vi "CSHostTest.vi"() -> ()   [LabVIEW 2014]
uses:
  <vilib>/FPGAPlugInAG/PXI-7852R/niLvFpga_Open_PXI-7852R.vi
  <vilib>/rvi/interface/common/dynamic/niFpgaDynamicAddResources.vi
  <vilib>/rvi/interface/common/niFpgaWaitOnOcc.vi
  <vilib>/Utility/error.llb/Error Cluster From Error Code.vi
  <vilib>/rvi/errors/niLvFpgaAdjustHostInterfaceError.vi
  <vilib>/FPGAPlugInAG/Dynamic/niLvFpga_Close_Dynamic.vi
  <vilib>/rvi/interface/nirviOpenFPGA/nirviOpenFPGA.xnode
  FPGA Bitfiles/TiTaProj_DAF_sequencerCWTopLevel_102.lvbitx
  <vilib>/rvi/interface/nirviMethod/nirviMethod.xnode
  <vilib>/rvi/interface/nirviReadWriteControl/nirviReadWriteControl.xnode
  <vilib>/rvi/interface/nirviCloseFPGA/nirviCloseFPGA.xnode
  <vilib>/rvi/interface/Simulation/niFpgaSimulationCallBeginRW.vi
  <vilib>/FPGAPlugInAG/Dynamic/niLvFpga_ReadFifo_Dynamic.vi
  <vilib>/rvi/errors/niLvFpgaMergeErrorWithErrorCode.vi
  NiFpgaLv.dll
  <vilib>/FPGAPlugInAG/Dynamic/niLvFpga_ConfigureFifo_Dynamic.vi
panel:
  in  "SendCommand":bool
  out "SavedData":u32[](array[numeric]) format="%032b"
  out "CounterArray":u32[][][](array[numeric])
  out "VoltArray":u32[](array[numeric]) format="%032b"
  in  "AnalyseData":bool
  in  "dwellTime":u32=2000000
  out "ReadData":u32[](array[numeric]) format="%032b"
  in  "stop":bool
  in  "abort":bool
  in  "hostConfirmsHzOffsetIsSet":bool
  in  "halt":bool
  in  "SetParameters":bool
  in  "VoltOrScaler?":bool
  in  "stepSize":i32=32768 format="%024b"
  in  "start":i32 format="%024b"
  in  "nOfSteps":i32=20
  in  "nOfScans":i32=6
  in  "invertScan":bool
  in  "heinzingerControl":T1(ring)
  in  "waitForKepco(25nsTicks)":u16
  in  "waitAfterReset(25nsTicks)":u16
  in  "measVoltPulseLength(25ns)":i32
  in  "measVoltTimeout(10ns)":i32
  in  "cmdByHost":T2(ring)
  out "measVoltState":T3(ring)
  out "seqState":T2(ring)
  out "SCstate":enum16{"idle", "scanning", "done", "error"}(ring)
  out "SCerrorcount":u8
  out "DACQuWriteTimeout":bool
  out "SCQuWriteTimeout":bool
  # "Scan"
  # "nOfPMT"
  # "Step"
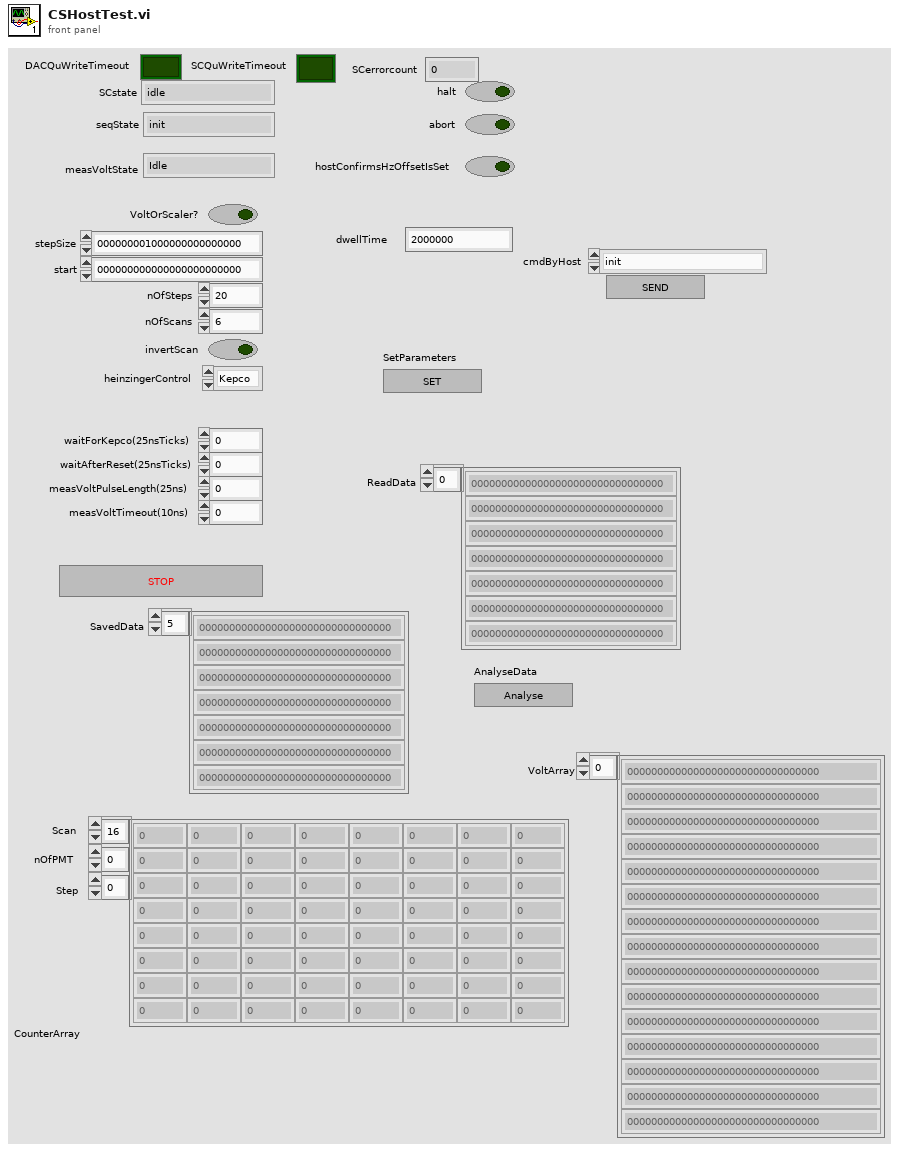
[diagram p1: front panel]
types:
  T1 = enum8{"Kepco", "Heinzinger0", "Heinzinger1", "Heinzinger2"}
  T2 = enum16{"init", "idle", "measureOffset", "measureTrack", "measComplete", "error"}
  T3 = enum16{"Idle", "sendMeasRequest", "waitUntilDone", "done"}
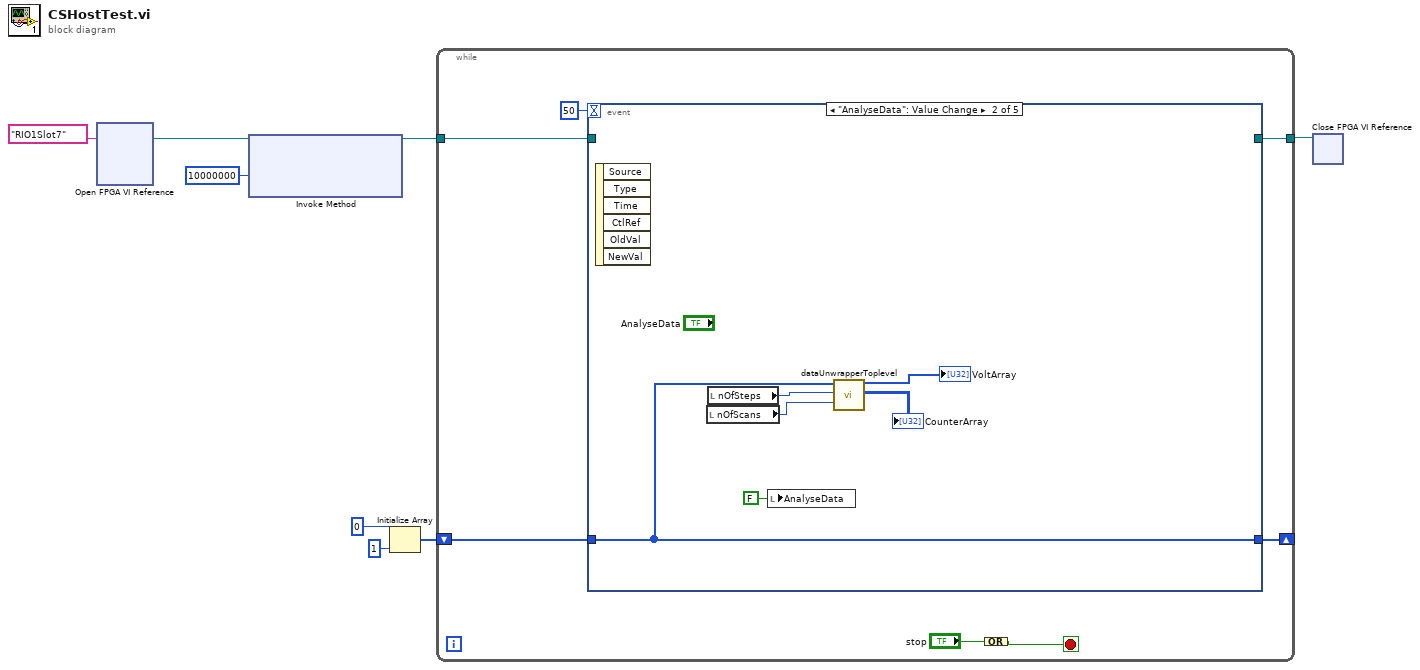
[diagram p0: block diagram]
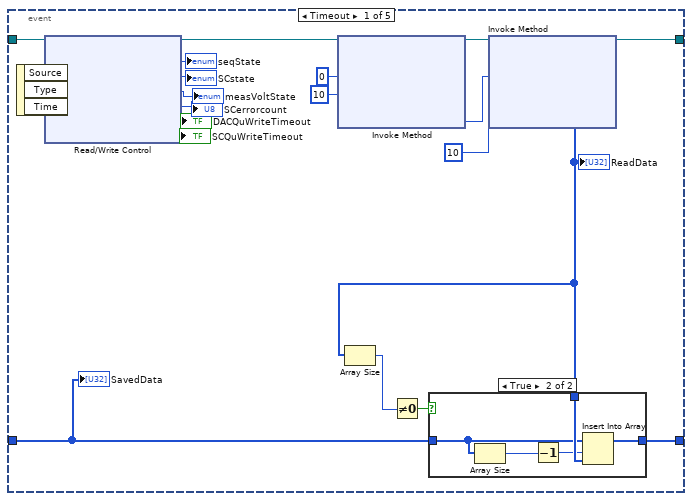
[diagram p2: hidden frame]
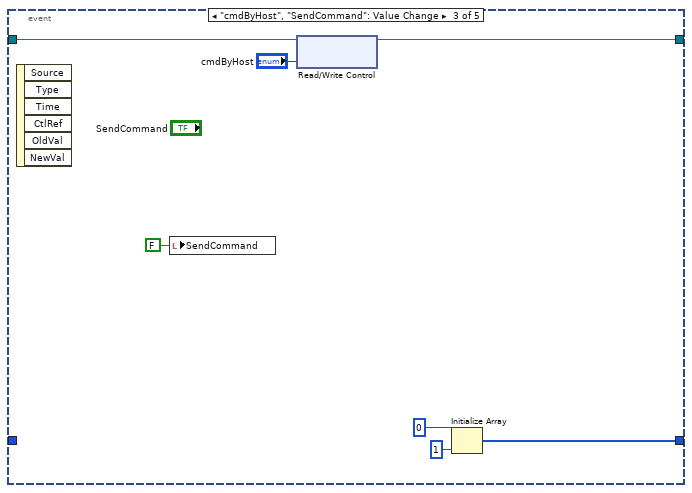
[diagram p4: hidden frame]
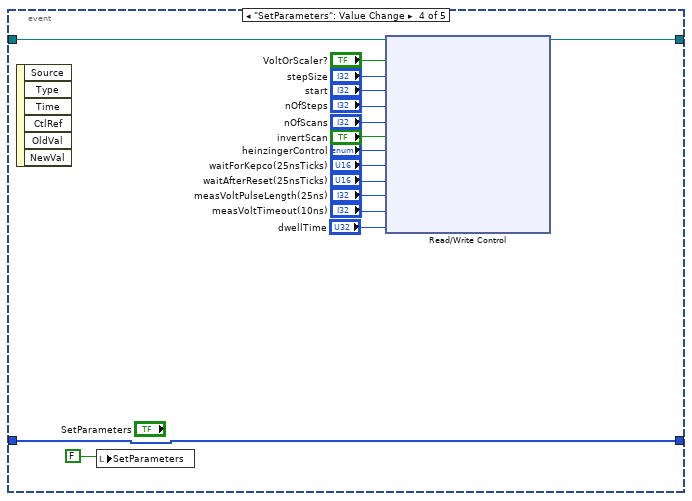
[diagram p5: hidden frame]
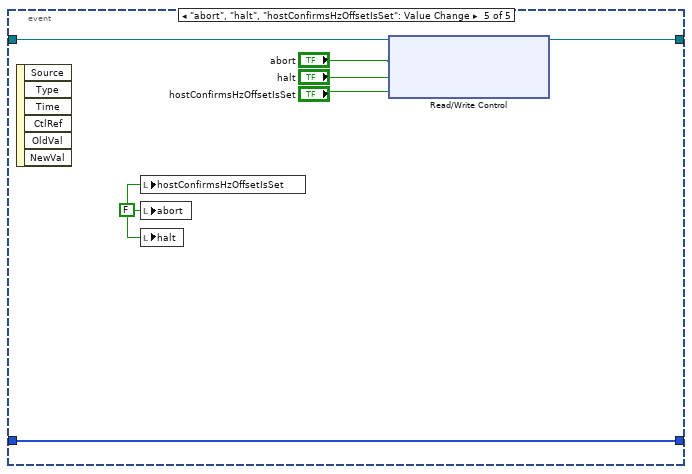
[diagram p6: hidden frame]
diagram:
  n1 = xnode "Open FPGA VI Reference"("resource name"=tag "RIO1Slot7") -> ("FPGA VI Reference Out"=w8:refnum<k20>)  [unwired: 1 in, 1 out]
  n2 = xnode "Invoke Method"("FPGA VI Reference In"=w8, "Requested Depth"=u32 10000000) -> ("FPGA VI Reference Out"=w5:refnum<k20>)  [unwired: 1 in, 2 out]
  n3 = Initialize Array(u32 0 ("element"), 1 ("dimension size")) -> (w3:u32[])
  n4 = while {
    tunnel: w5 -> [w12]
    tunnel: [w11] -> w7
    shift-right: [w10] -> _
    shift-left: w3 -> [w9]
    stop <- w13 stop-if-true
    n5 = event shown="[1] \"AnalyseData\": Value Change" {
      selector: _ -> [_ _ _ _ _]
      dyn-events: _ -> [_ _ _ _ _]
      timeout: 50 -> [_ _ _ _ _]
      tunnel: w12 -> [w34 _ w53 w68 w75]
      tunnel: [w28 _ w52 w56 w74] -> w11
      tunnel: [w21 w46 w48 w54 w70] -> w10
      tunnel: w9 -> [w16 w46 _ w54 w70]
      event Timeout {
        n6 = event-data() -> ()  [unwired: 1 in, 3 out]
        n7 = xnode "Read/Write Control"("FPGA VI Reference In"=w34) -> ("FPGA VI Reference Out"=w32:refnum<k20>, "seqState"=→"seqState":T2, "SPstate"=→"SCstate":enum16{"idle", "scanning", "done", "error"}, "measVoltState"=→"measVoltState":T3, "SPerrorCount"=→"SCerrorcount":u8, "DACQuWriteTimeout"=→"DACQuWriteTimeout":bool, "SPCtrQuWriteTimeout"=→"SCQuWriteTimeout":bool)  [unwired: 1 in, 1 out]
        n8 = xnode "Invoke Method"("FPGA VI Reference In"=w32, "Number of Elements"=u32 0, "Timeout (ms)"=10) -> ("FPGA VI Reference Out"=w31:refnum<k20>, "Elements Remaining"=w19:u32)  [unwired: 1 in, 2 out]
        n9 = xnode "Invoke Method"("FPGA VI Reference In"=w31, "Number of Elements"=w19, "Timeout (ms)"=10) -> ("FPGA VI Reference Out"=w28:refnum<k20>, "Data"=w17:u32[])  [unwired: 1 in, 2 out]
        "ReadData" <- w17
        n10 = Array Size(array=w17) -> (size(s)=w18:i32)
        n11 = Not Equal To 0?(x=w18) -> (x != 0?=w20:bool)
        n12 = case shown="True" w20 {
          tunnel: w17 -> [_ w40]
          tunnel: [w35 w39] -> w21
          tunnel: w16 -> [w35 w38]
          frame False {
          }
          frame True {
            n13 = Array Size(array=w38) -> (size(s)=w37:i32)
            n14 = Decrement(x=w37) -> (x-1=w36:i32)
            n15 = Insert Into Array(array=w38, index=w36, new element=w40) -> (w39:u32[])
          }
        }
        "SavedData" <- w16
      }
      event "AnalyseData": Value Change {
        n16 = event-data() -> ()  [unwired: 1 in, 6 out]
        n17 = local read "nOfScans"() -> (w44:i32)
        n18 = local read "nOfSteps"() -> (w45:i32)
        n19 = local write "AnalyseData"(FALSE ("AnalyseData")) -> ()
        n20 = call "dataUnwrapperToplevel.vi"("SCdata"=w46, "nOfSteps"=w45, "nOfScans"=w44) -> ("VoltArray"=→"VoltArray":u32[], "CounterArray"=→"CounterArray":u32[][][])  [unwired: 15 in]
      }
      event "cmdByHost", "SendCommand": Value Change {
        n21 = event-data() -> ()  [unwired: 1 in, 6 out]
        n22 = local write "SendCommand"(FALSE ("SendCommand")) -> ()
        n23 = xnode "Read/Write Control"("FPGA VI Reference In"=w53, "cmdByHost"="cmdByHost") -> ("FPGA VI Reference Out"=w52:refnum<k20>)  [unwired: 1 in, 1 out]
        n24 = Initialize Array(u32 0 ("element"), 1 ("dimension size")) -> (w48:u32[])
      }
      event "SetParameters": Value Change {
        n25 = event-data() -> ()  [unwired: 1 in, 6 out]
        n26 = local write "SetParameters"(FALSE ("SetParameters")) -> ()
        n27 = xnode "Read/Write Control"("FPGA VI Reference In"=w68, "VoltOrScaler?"="VoltOrScaler?", "stepSize"="stepSize", "start"="start", "nOfSteps"="nOfSteps", "nOfScans"="nOfScans", "invertScan"="invertScan", "heinzingerControl"="heinzingerControl", "waitForKepco(25nsTicks)"="waitForKepco(25nsTicks)", "waitAfterReset(25nsTicks)"="waitAfterReset(25nsTicks)", "measVoltPulseLength(25ns)"="measVoltPulseLength(25ns)", "measVoltTimeout(10ns)"="measVoltTimeout(10ns)", "dwellTime"="dwellTime") -> ("FPGA VI Reference Out"=w56:refnum<k20>)  [unwired: 1 in, 1 out]
      }
      event "abort", "halt", "hostConfirmsHzOffsetIsSet": Value Change {
        w76 = FALSE ("abort")
        n28 = event-data() -> ()  [unwired: 1 in, 6 out]
        n29 = local write "hostConfirmsHzOffsetIsSet"(w76) -> ()
        n30 = local write "abort"(w76) -> ()
        n31 = local write "halt"(w76) -> ()
        n32 = xnode "Read/Write Control"("FPGA VI Reference In"=w75, "abort"="abort", "halt"="halt", "hostConfirmsHzOffsetIsSet"="hostConfirmsHzOffsetIsSet") -> ("FPGA VI Reference Out"=w74:refnum<k20>)  [unwired: 1 in, 1 out]
      }
    }
    n33 = Compound Arithmetic op=OR("stop") -> (w13:bool)
  }
  n34 = xnode "Close FPGA VI Reference"("FPGA VI Reference In"=w7) -> ()  [unwired: 1 in, 1 out]
